vi "Agilent34410A Set TrigSource.vi"(8 "error in (no error)":errorcluster, 10 "Trigger Source":enum16{"Immediate", "External", "Bus"}(ring), 11 "VISA Rsrc":refnum<visa-resource-name>="SR530") -> (0 "error out":errorcluster, 3 "VISA Rsrc Out":refnum<visa-resource-name>="GPIB0::12::INSTR", 4 "ChaineCom":string caption="Chaîne de commande")   [LabVIEW 2019]
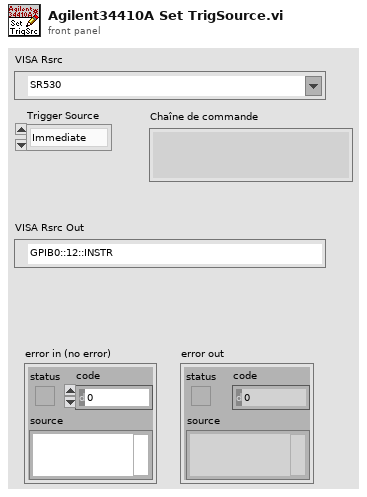
[diagram p1: front panel]
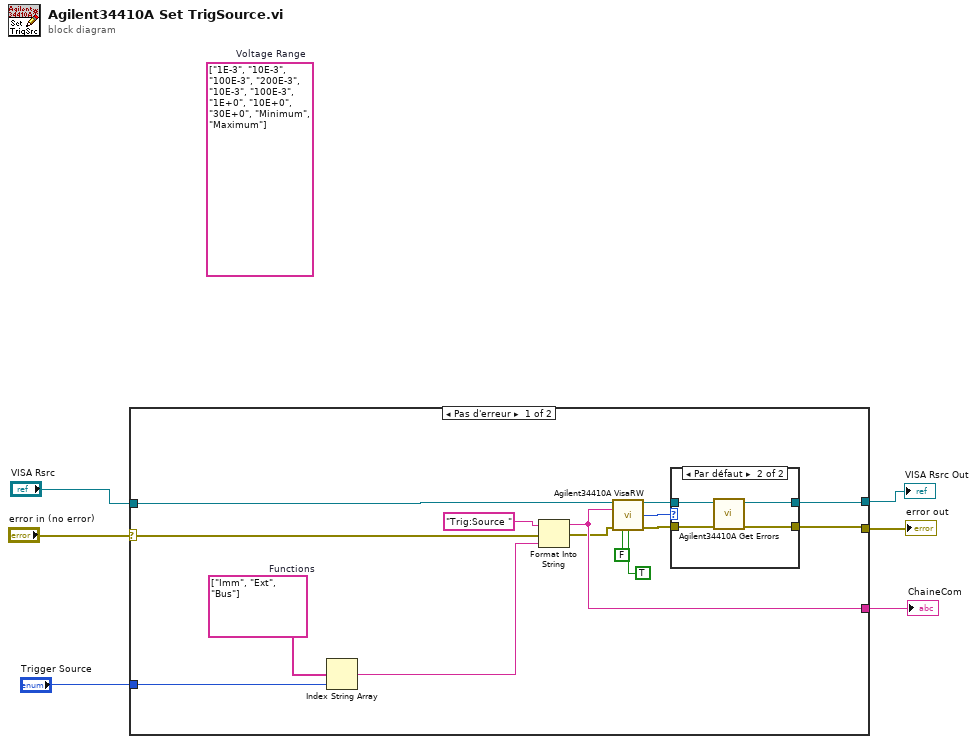
[diagram p0: block diagram]
diagram:
  (unwired) string[] ["1E-3", "10E-3", "100E-3", "200E-3", "10E-3", "100E-3", "1E+0", "10E+0", "30E+0", "Minimum", "Maximum"]  # Voltage Range
  n1 = case shown="Pas d'erreur" "error in (no error)" {
    selector: "error in (no error)" -> [w19 w28]
    tunnel: "VISA Rsrc" -> [w21 w29]
    tunnel: [w18 w28] -> w4
    tunnel: [w17 w29] -> w3
    tunnel: [w20 _] -> w2
    tunnel: "Trigger Source" -> [w16 _]
    frame No Error {
      w15 = string[] ["Imm", "Ext", "Bus"]  # Functions
      n2 = Index String Array(1:w16, 2:w15) -> (0:w8:string)  [unwired: 1 in]
      n3 = Format Into String(initial string="Trig:Source " ("string (\"\")"), error in=w19, w8) -> (resulting string=w20:string, error out=w12:errorcluster)  [unwired: 1 in]
      n4 = call <userlib>:"Agilent34410A VisaRW.vi"("VISA Rsrc"=w21, "ChaineCom"=w20, "error in (no error)"=w12, "Lecture?(T)"=FALSE, "Poll?(F)"=TRUE) -> ("VISA Rsrc Out"=w11:refnum<visa-resource-name>, "octet d'état"=w10:u16, "error out"=w9:errorcluster)  [unwired: 6 in, 2 out]
      n5 = case shown="Par défaut" w10 {
        tunnel: w11 -> [w23 w27]
        tunnel: w9 -> [w22 w26]
        tunnel: [w22 w25] -> w18
        tunnel: [w23 w24] -> w17
        frame 0 {
        }
        frame Default {
          n6 = call <userlib>:"Agilent34410A Get Errors.vi"("error in (no error)"=w26, "VISA Rsrc"=w27) -> ("error out"=w25:errorcluster, "VISA Rsrc Out"=w24:refnum<visa-resource-name>)  [unwired: 7 in, 1 out]
        }
      }
    }
    frame Error {
    }
  }
  "error out" <- w4
  "VISA Rsrc Out" <- w3
  "ChaineCom" <- w2
